vi "Test2_3b_ASIC_mezzanine_pepe.vi"(0 "Instrument VISA in":T1={"AWG VISA"="generadorpulsos", "Oscilloscope  VISA "="Oscilloscope", "Integration Board IP"="172.16.7.43", "connection ID"=refnum, "report out"=refnum, "report file path"=path "D:/CTA/Data_test/ASIC/test3a"}, 5 "quantity":i32=3, 7 "Cycles Burst":i32=10000, 9 "L1 Address":i32=17, 11 "error in":errorcluster={"status"=FALSE, "code"=0, "source"="VISA Write in Test2_3a_ASIC_fast.vi->test_sum_ASIC.vi"}, 12 "channel array":i32[](array[numeric])=[0, 1, 2, 3, 4, 5, 6]) -> (4 "Instrument VISA out":T1={"AWG VISA"="generadorpulsos", "Oscilloscope  VISA "="Oscilloscope", "Integration Board IP"="172.16.7.43", "connection ID"=refnum, "report out"=refnum, "report file path"=path "D:/CTA/Data_test/test3a"}, 15 "error out":errorcluster)   [LabVIEW 2009]
uses:
  <vilib>/Utility/NIReport.llb/NI_report.lvclass
  <vilib>/Utility/NIReport.llb/HTML/NI_HTML.lvclass
  <instrlib>/Agilent 8000 Series/Public/Configure/Configure Math (Binary Operation).vi
  <instrlib>/Agilent 81150/Agilent 81150.lvlib
  L0_Asic/L0 Asic Test Folder v9/C/Program Files/National Instruments/LabVIEW 2012/instr.lib/Agilent 8000 Series/Agilent 8000 Series.lvlib
panel:
  in  "Cycles Burst 2":i32=10000
  out "Filename Out":path
  out "appended path":path
  out "Array":i32[](array[numeric])=[2, 3, 5]
  out "points quantity":dbl=94.0
  out "appended array":dbl[](array[numeric])=[0.75, 42.0, 0.0, 63.0, 1.0, 1.069, 0.0055, 2.925838e-09, 1.2702e-11, 0.0555, 0.0035, 9.99999e+37, 9.99999e+37, 6.264189e-09, 3.2805e-11, 94.0]
  out "read buffer 3":string="V amptd(f2),1.074E+00,0,1.056E+00,1.087E+00,1.0690E+00,5.5E-03,9.4E+01,+ width(f2),2.90015E-09,0,2.90015E-09,2.95960E-09,2.925838E-09,1.2702E-11,9.4E+01,V amptd(1),5.5E-02,0,4.8E-02,6.7E-02,5.55E-02,3.5E-03,9.4E+01,+ width(f1),9.99999E+37,5,9.99999E+37,9.99999E+37,9.99999E+37,9.99999E+37,9.99999E+37,Time(f1-f2),6.26722E-09,0,6.20145E-09,6.35270E-09,6.264189E-09,3.2805E-11,9.4E+01\n"
  in  "Quantity of measurements":u32=100
  in  "Voltage":dbl[](array[numeric])=[0.05, 0.2, 0.5, 0.7, 1.0]
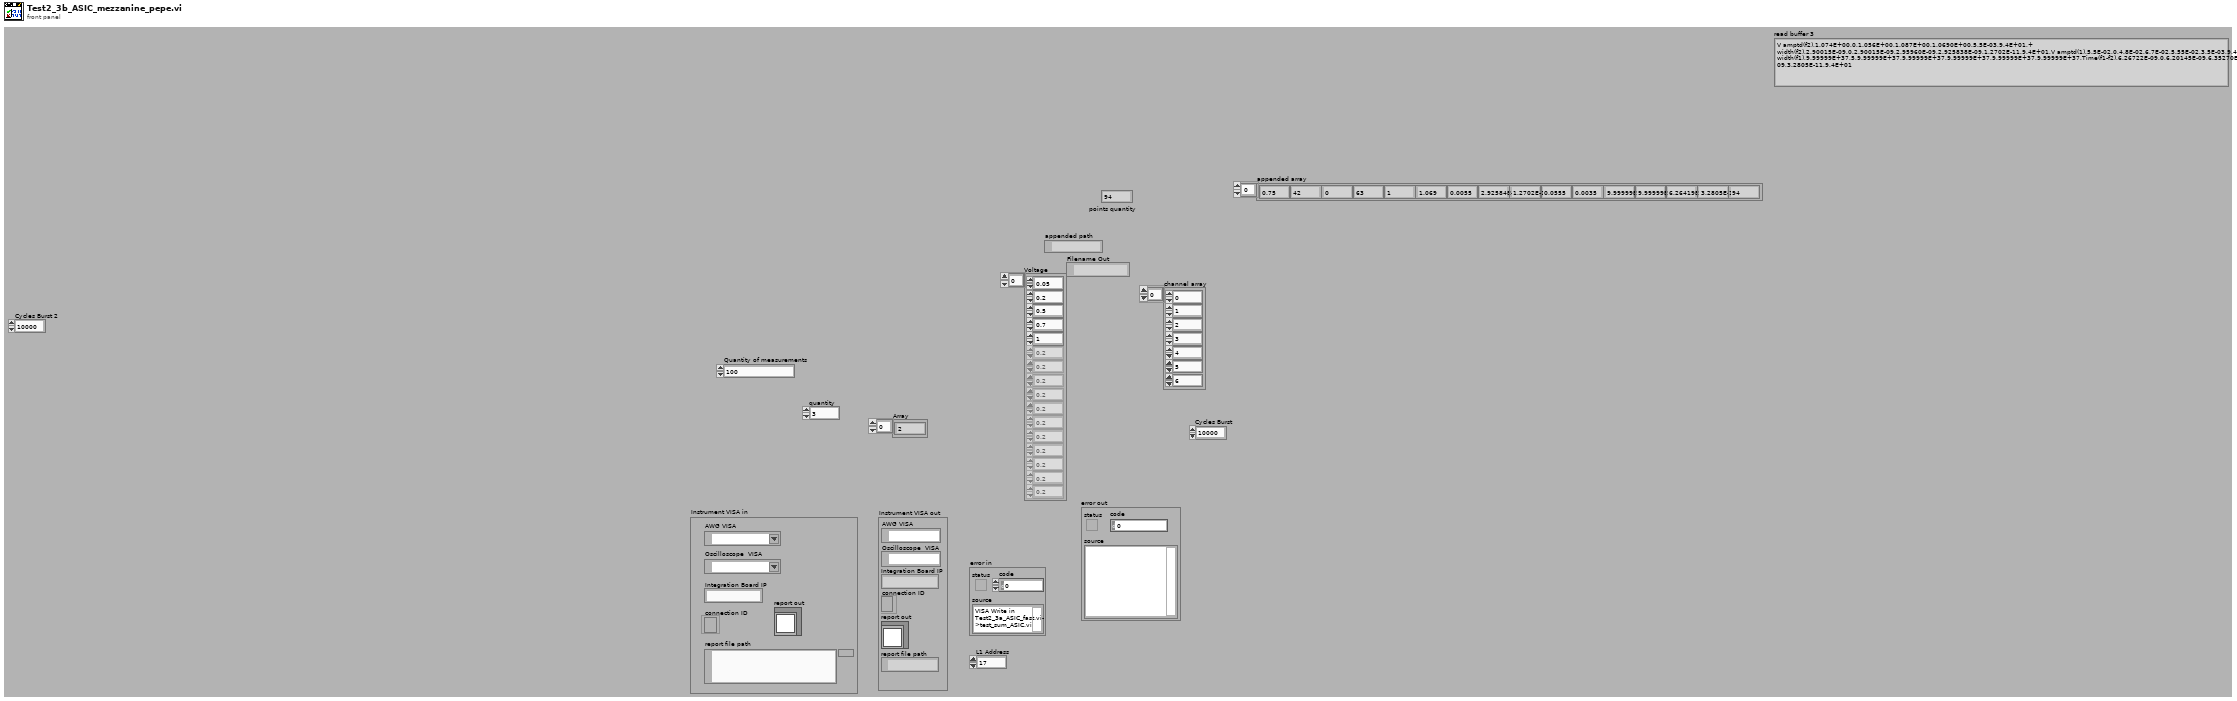
[diagram p1: front panel]
types:
  T1 = cluster{"AWG VISA":refnum<visa-resource-name>, "Oscilloscope  VISA ":refnum<visa-resource-name>, "Integration Board IP":string, "connection ID":refnum<k5>, "report out":refnum<class "NI_report.lvclass">, "report file path":path}
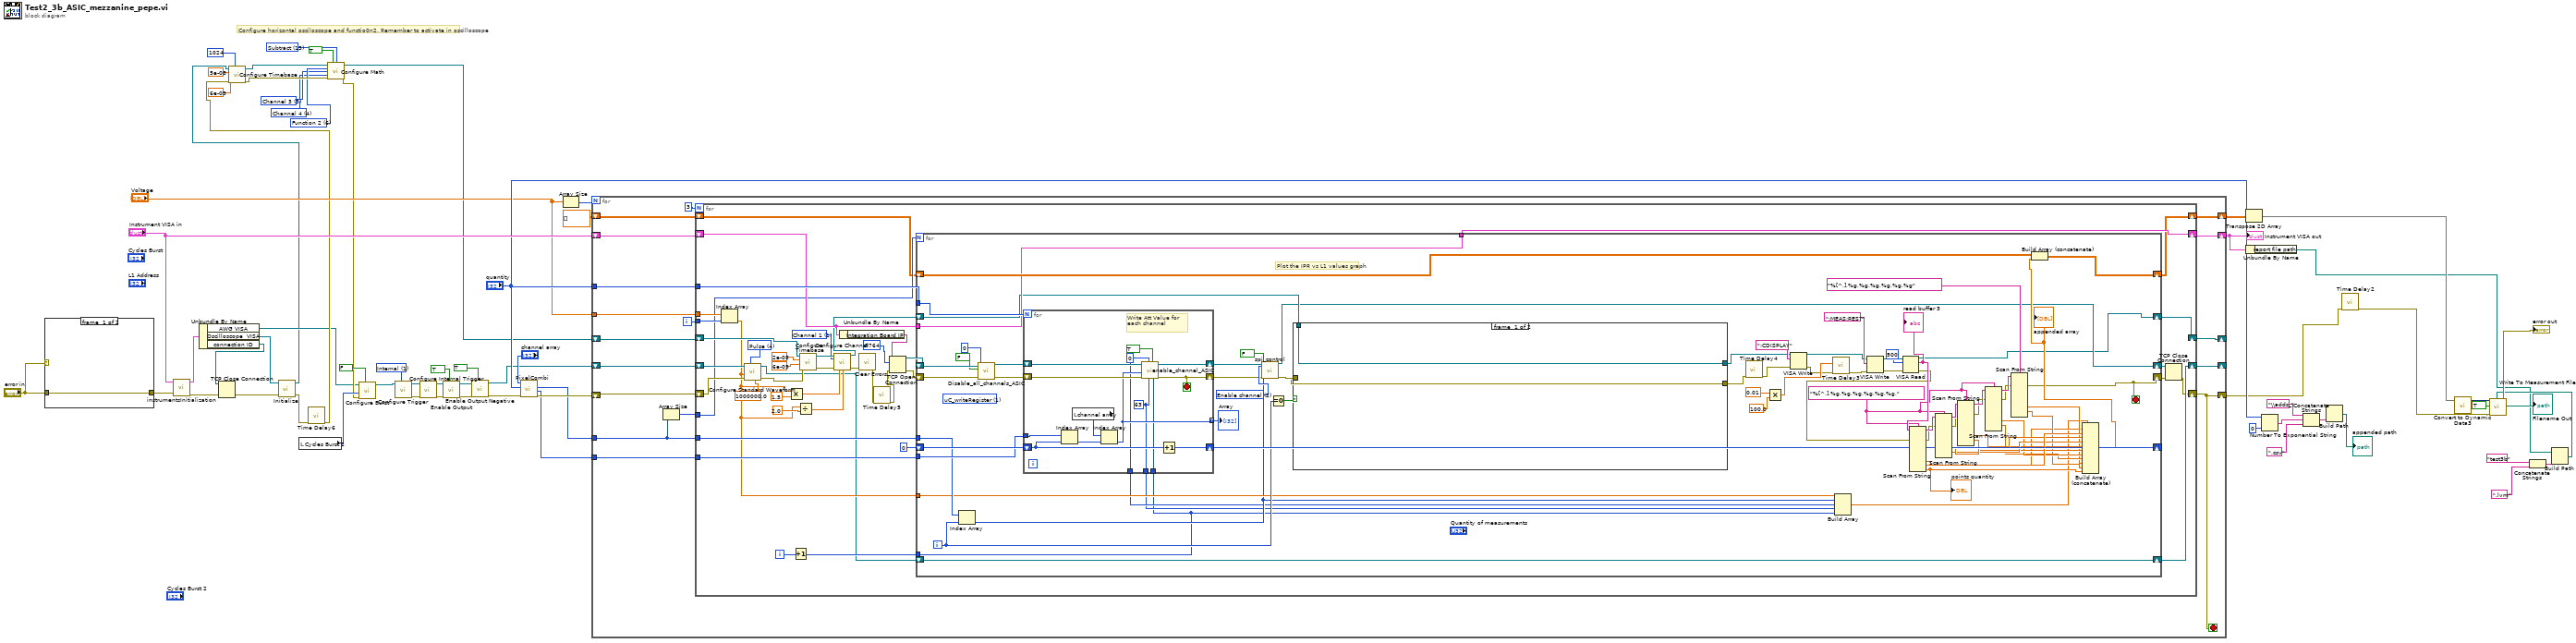
[diagram p0: block diagram]
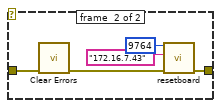
[diagram p2: hidden frame]
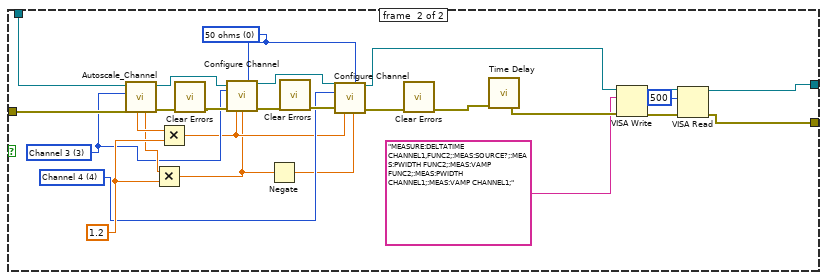
[diagram p3: hidden frame]
diagram:
  w13 = u16 6 items=["Function 1"=5, "Function 2"=6, "Function 3"=7, "Function 4"=8] ("Math Channel (5: Function 1)")
  w17 = u16 15 items=["Add"=12, "Divide"=13, "Multiply"=14, "Subtract"=15, "Common Mode"=16, "Versus"=17] ("Math Operation (12: Add)")
  w12 = 3 items=["Channel 1"=1, "Channel 2"=2, "Channel 3"=3, "Channel 4"=4] ("Channel (1: Channel 1)")
  w11 = 4 items=["Channel 1"=1, "Channel 2"=2, "Channel 3"=3, "Channel 4"=4] ("Channel (1: Channel 1)")
  w40 = u16 1 items=["Immediate", "Internal", "External", "Software Trigger Function"] ("Trigger Source (0: Immediate)")
  # "Configure horizontal osciloscope and functio0n2. Remember to activate in oscilloscope"
  n1 = case shown="No Error" "error in" {
    tunnel: "error in" -> [w66 w68]
    tunnel: [w66 w71] -> w36
    frame #0 {
    }
    frame #1 {
      n2 = call <vilib>:"Clear Errors.vi"("error in (no error)"=w68) -> ("error out"=w67:errorcluster)  [unwired: 6 in]
      n3 = call "resetboard.vi"("error in (no error)"=w67, "address"="172.16.7.43", "remote port or service name"=u16 9764) -> ("error out"=w71:errorcluster)  [unwired: 7 in, 1 out]
    }
  }
  n4 = call "instrumentsInitialization.vi"("error in"=w36, "Instrument VISA in"="Instrument VISA in") -> ("error out"=w27:errorcluster, "Instrument VISA out"=w58:T1)  [unwired: 8 in]
  n5 = Unbundle By Name(w58) -> ("AWG VISA"=w4:refnum<visa-resource-name>, "Oscilloscope  VISA"=w26:refnum<visa-resource-name>, "connection ID"=w35:refnum<k5>)
  n6 = TCP Close Connection(connection ID=w35) -> ()  [unwired: 2 in, 2 out]
  n7 = call <instrlib>:"Initialize.vi"("error in (no error)"=w27, "VISA resource name"=w26) -> ("error out"=w7:errorcluster, "VISA resource name out"=w1:refnum<visa-resource-name>)  [unwired: 8 in]
  n8 = local read "Cycles Burst 2"() -> (w8:i32)
  n9 = call "Time Delay6"("error in (no error)"=w7) -> ("error out"=w6:errorcluster)  [unwired: 10 in]
  n10 = call <instrlib>:"Configure Timebase.vi"("Record Length (1000)"=1024, "error in (no error)"=w6, "Position (0.0 s)"=6e-09, "Timebase (0.005 s)"=5e-08, "VISA resource name"=w1) -> ("error out"=w14:errorcluster, "VISA resource name out"=w15:refnum<visa-resource-name>)  [unwired: 5 in]
  n11 = call-poly <instrlib>:"Configure Math.vi"("VISA resource name"=w15, "Enable Math Channel (T:Enable)"=TRUE, "Math Operation (12: Add)"=w17, "Math Channel (5: Function 1)"=w13, "Math Operand (1: Channel 1)"=w12, "Math Operand (2: Channel 2)"=w11, "error in (no error)"=w14) -> ("VISA resource name out"=w2:refnum<visa-resource-name>, "error out"=w5:errorcluster)  [unwired: 7 in]
  n12 = call <instrlib>:"Configure Burst.vi"("Enable Burst (F: Disable)"=FALSE, "error in (no error)"=w5, "Burst Count (2)"=w8, "VISA resource name"=w4) -> ("VISA resource name out"=w3:refnum<visa-resource-name>)  [unwired: 6 in, 1 out]
  n13 = call <instrlib>:"Configure Trigger.vi"("Trigger Source (0: Immediate)"=w40, "VISA resource name"=w3) -> ("error out"=w41:errorcluster, "VISA resource name out"=w42:refnum<visa-resource-name>)  [unwired: 8 in]
  n14 = call <instrlib>:"Configure Internal Trigger.vi"("error in (no error)"=w41, "VISA resource name"=w42) -> ("error out"=w43:errorcluster, "VISA resource name out"=w44:refnum<visa-resource-name>)  [unwired: 8 in]
  n15 = call <instrlib>:"Enable Output.vi"("Enable Output (T: Enable)"=TRUE, "error in (no error)"=w43, "VISA resource name"=w44) -> ("error out"=w34:errorcluster, "VISA resource name out"=w33:refnum<visa-resource-name>)  [unwired: 7 in]
  n16 = call <instrlib>:"Enable Output Negative.vi"("Enable Output (T: Enable)"=TRUE, "error in (no error)"=w34, "VISA resource name"=w33) -> ("error out"=w32:errorcluster, "VISA resource name out"=w31:refnum<visa-resource-name>)  [unwired: 7 in]
  n17 = call "PixelCombi.vi"("error in"=w32, "quantity"="quantity", "array"="channel array") -> ("error out"=w64:errorcluster, "Channels"=w63:i32[], "Combination Array"=w62:i16[])  [unwired: 6 in]
  n18 = Array Size(array="Voltage") -> (size(s)=w59:i32)
  n19 = for {
    N: w59 -> [_]
    tunnel: w63 -> [w86]
    tunnel: w62 -> [w85]
    shift-right: [w72] -> w46
    shift-left: w64 -> [w88]
    tunnel: "Voltage" -> [w84]
    tunnel: "quantity" -> [w82]
    shift-right: [w77] -> w45
    shift-left: "Instrument VISA in" -> [w80]
    shift-right: [w76] -> w49
    shift-left: dbl[][] [] -> [w78]
    shift-right: [w73] -> _
    shift-left: w31 -> [w87]
    shift-right: [w74] -> _
    shift-left: w2 -> [w81]
    i -> [w83]
    stop <- w72 stop-if-true
    n20 = Array Size(array=w85) -> (size(s)=w79:i32)
    n21 = for {
      N: 3 -> [_]
      tunnel: w86 -> [w127]
      tunnel: w85 -> [w125]
      tunnel: w84 -> [w124]
      tunnel: w83 -> [w123]
      tunnel: w82 -> [w122]
      tunnel: w79 -> [w107]
      shift-right: [w97] -> w76
      shift-left: w78 -> [w100]
      shift-right: [w98] -> w77
      shift-left: w80 -> [w111]
      shift-right: [w92] -> w72
      shift-left: w88 -> [w129]
      shift-right: [w93] -> w73
      shift-left: w87 -> [w128]
      shift-right: [w95] -> w74
      shift-left: w81 -> [w118]
      i -> [w89]
      w114 = 1 items=["Channel 1"=1, "Channel 2"=2, "Channel 3"=3, "Channel 4"=4] ("Channel (1: Channel 1)")
      w131 = u16 4 items=["Sine", "Square", "Ramp Up", "Ramp Down", "Pulse", "Noise", "DC"] ("Waveform (0: Sine)")
      n22 = Index Array(array=w124, index=w123) -> (element=w99:dbl)
      n23 = call <instrlib>:"Configure Standard Waveform.vi"("Frequency (1000.0 Hz)"=1000000.0, "Waveform (0: Sine)"=w131, "error in (no error)"=w129, "Amplitude (1.0 Vpp)"=w99, "VISA resource name"=w128) -> ("error out"=w121:errorcluster, "VISA resource name out"=w94:refnum<visa-resource-name>)  [unwired: 5 in]
      n24 = Multiply(x=w99, y=1.5) -> (x*y=w113:dbl)
      n25 = Increment(x=w89) -> (x+1=w96:i32)
      n26 = Divide(x=w99, y=2.0) -> (x/y=w105:dbl)
      n27 = call <instrlib>:"Configure Timebase.vi"("error in (no error)"=w121, "Position (0.0 s)"=6e-09, "Timebase (0.005 s)"=2e-08, "VISA resource name"=w118) -> ("error out"=w120:errorcluster, "VISA resource name out"=w117:refnum<visa-resource-name>)  [unwired: 6 in]
      n28 = call "Configure Channel.vi"("VISA resource name"=w117, "Channel (1: Channel 1)"=w114, "error in (no error)"=w120, "Vertical Range (2.0 V)"=w113, "Vertical Offset (0.0 V)"=w105) -> ("VISA resource name out"=w104:refnum<visa-resource-name>, "error out"=w119:errorcluster)  [unwired: 9 in]
      n29 = Unbundle By Name(w111) -> ("Integration Board IP"=w109:string)
      n30 = call <vilib>:"Clear Errors.vi"("error in (no error)"=w119) -> ("error out"=w91:errorcluster)  [unwired: 6 in]
      n31 = call "Time Delay5"("error in (no error)"=w91) -> ("error out"=w90:errorcluster)  [unwired: 10 in]
      n32 = TCP Open Connection(address=w109, remote port or service name=u16 9764, error in (no error)=w90) -> (connection ID=w101:refnum<k5>, error out=w110:errorcluster)  [unwired: 2 in]
      n33 = for {
        N: w107 -> [_]
        tunnel: w125 -> [w199]
        tunnel: w127 -> [w200]
        shift-right: [w201] -> _
        shift-left: i16 0 ("element") -> [w202]
        shift-right: [w146] -> w103
        shift-left: w110 -> [w192]
        tunnel: w111 -> [w187]
        tunnel: w122 -> [w198]
        tunnel: [w187] -> w98
        shift-right: [w193] -> w97
        shift-left: w100 -> [w194]
        shift-right: [w147] -> w102
        shift-left: w101 -> [w145]
        tunnel: w99 -> [w142]
        tunnel: w96 -> [w137]
        shift-right: [w136] -> w95
        shift-left: w104 -> [w185]
        shift-right: [w135] -> w93
        shift-left: w94 -> [w135]
        i -> [w183]
        stop <- w146 stop-if-true
        w168 = "%[^,],%g,%g,%g,%g,%g,%g," ("format string")
        w191 = u16 2 items=["Attenuation", "Clipping", "Enable channel", "Delay line", "ASIC"] ("Device")
        (unwired) u16 1 items=["sendCommand"=9, "FPGA_writeRegister"=3, "FPGA_readRegister"=2, "uC_writeRegister"=1, "uC_readRegister"=0] ("Action")
        # "Plot the IPR vs L1 values graph"
        n34 = Index Array(array=w199, index=w183) -> (element=w141:i16)
        n35 = call "Disable_all_channels_ASIC.vi"("error in"=w192, "id_in"=0 ("Data"), "Clip_en_b"=FALSE, "connection ID"=w145) -> ("error out"=w196:errorcluster, "connection ID out"=w195:refnum<k5>)  [unwired: 5 in, 1 out]
        n36 = for {
          N: w198 -> [_]
          shift-right: [w244] -> w201
          shift-left: w202 -> [w245]
          tunnel: w200 -> [w243]
          shift-right: [w240] -> w189
          shift-left: w196 -> [w239]
          shift-right: [w237] -> w188
          shift-left: w195 -> [w238]
          tunnel: [w236] -> w144 mode=indexing
          tunnel: [w235] -> w140
          tunnel: [w234] -> w139
          tunnel: w137 -> [w233]
          stop <- w240 stop-if-true
          w235 = u32 0 ("Att gain")
          w234 = u32 63 ("Ib_clipVb")
          # "Write Att Value for each channel"
          n37 = Index Array(array=w243, index=w245) -> (element=w241:i32)
          n38 = local read "channel array"() -> (w242:i32[])
          n39 = Index Array(array=w242, index=w241) -> (element=w236:i32)
          n40 = call "enable_channel_ASIC.vi"("Clip_sel_b"=w233, "maj/sum"=TRUE, "Ib_clipVb"=w234, "Att gain"=w235, "error in"=w239, "Channel"=w236, "connection ID"=w238) -> ("error out"=w240:errorcluster, "connection ID out"=w237:refnum<k5>)  [unwired: 2 in, 1 out]
          n41 = Increment(x=w245) -> (x+1=w244:i16)
        }
        "Array" <- w144
        n42 = call "spi_control.vi"("connection ID"=w188, "Device"=w191, "Read/#write"=FALSE, "Data"=w141, "error out 3"=w189) -> ("connection ID out"=w147:refnum<k5>, "error out 2"=w186:errorcluster)  [unwired: 7 in, 6 out]
        n43 = Equal To 0?(x=w183) -> (x = 0?=w184:bool)
        n44 = case shown="True" w184 {
          tunnel: [w204 w211] -> w132
          tunnel: w186 -> [w204 w217]
          tunnel: w185 -> [w203 w218]
          tunnel: [w203 w220] -> w150
          frame #0 {
          }
          frame #1 {
            w221 = u32 0 items=["50 ohms", "1 Mohms"] ("Input Impedance (1: 1 Mohms)")
            w209 = 3 items=["Channel 1"=1, "Channel 2"=2, "Channel 3"=3, "Channel 4"=4] ("Channel (1: Channel 1)")
            w208 = 4 items=["Channel 1"=1, "Channel 2"=2, "Channel 3"=3, "Channel 4"=4] ("Channel (1: Channel 1)")
            w214 = 1.2 ("y")
            n45 = call "Autoscale_Channel.vi"("error in"=w217, "Channel"=w209, "VISA resource name"=w218) -> ("error out"=w228:errorcluster, "VISA resource name out"=w231:refnum<visa-resource-name>, "Offset"=w210:dbl, "VerticalRange"=w225:dbl)  [unwired: 5 in]
            n46 = Multiply(x=w210, y=w214) -> (x*y=w206:dbl)
            n47 = Multiply(x=w225, y=w214) -> (x*y=w207:dbl)
            n48 = call <vilib>:"Clear Errors.vi"("error in (no error)"=w228) -> ("error out"=w229:errorcluster)  [unwired: 6 in]
            n49 = call "Configure Channel.vi"("VISA resource name"=w231, "Input Impedance (1: 1 Mohms)"=w221, "Channel (1: Channel 1)"=w209, "error in (no error)"=w229, "Vertical Range (2.0 V)"=w207, "Vertical Offset (0.0 V)"=w206) -> ("VISA resource name out"=w226:refnum<visa-resource-name>, "error out"=w230:errorcluster)  [unwired: 8 in]
            n50 = Negate(x=w206) -> (-x=w205:dbl)
            n51 = call <vilib>:"Clear Errors.vi"("error in (no error)"=w230) -> ("error out"=w219:errorcluster)  [unwired: 6 in]
            n52 = call "Configure Channel.vi"("VISA resource name"=w226, "Input Impedance (1: 1 Mohms)"=w221, "Channel (1: Channel 1)"=w208, "error in (no error)"=w219, "Vertical Range (2.0 V)"=w207, "Vertical Offset (0.0 V)"=w205) -> ("VISA resource name out"=w215:refnum<visa-resource-name>, "error out"=w227:errorcluster)  [unwired: 8 in]
            n53 = call <vilib>:"Clear Errors.vi"("error in (no error)"=w227) -> ("error out"=w216:errorcluster)  [unwired: 6 in]
            n54 = call "Time Delay"("error in (no error)"=w216) -> ("error out"=w213:errorcluster)  [unwired: 10 in]
            n55 = VISA Write(VISA resource name=w215, write buffer="MEASURE:DELTATIME CHANNEL1,FUNC2;:MEAS:SOURCE?;:MEAS:PWIDTH FUNC2;:MEAS:VAMP FUNC2;:MEAS:PWIDTH CHANNEL1;:MEAS:VAMP CHANNEL1;", error in (no error)=w213) -> (VISA resource name out=w224:refnum<visa-resource-name>, error out=w223:errorcluster)  [unwired: 1 out]
            n56 = VISA Read(VISA resource name=w224, byte count=u32 500, error in (no error)=w223) -> (VISA resource name out=w220:refnum<visa-resource-name>, error out=w211:errorcluster)  [unwired: 2 out]
          }
        }
        n57 = call "Time Delay4"("error in (no error)"=w132) -> ("error out"=w133:errorcluster)  [unwired: 10 in]
        n58 = Multiply(x=0.01, y=100.0) -> (x*y=w175:dbl)
        n59 = VISA Write(VISA resource name=w150, write buffer=":CDISPLAY", error in (no error)=w133) -> (VISA resource name out=w153:refnum<visa-resource-name>, error out=w151:errorcluster)  [unwired: 1 out]
        n60 = call "Time Delay3"("error in (no error)"=w151, "Delay Time (s)"=w175) -> ("error out"=w174:errorcluster)  [unwired: 9 in]
        n61 = Build Array(w142, w141, w140, w139, w137) -> (w138:dbl[])
        n62 = VISA Write(VISA resource name=w153, write buffer=":MEAS:RES?", error in (no error)=w174) -> (VISA resource name out=w182:refnum<visa-resource-name>, error out=w181:errorcluster)  [unwired: 1 out]
        n63 = VISA Read(VISA resource name=w182, byte count=u32 500, error in (no error)=w181) -> (VISA resource name out=w136:refnum<visa-resource-name>, read buffer=w178:string, error out=w158:errorcluster)  [unwired: 1 out]
        "read buffer 3" <- w178
        n64 = Scan From String(format string=w168, input string=w178, error in=w158) -> (remaining string=w172:string, error out=w154:errorcluster, output 5=w143:dbl, output 6=w173:dbl, output 7=w159:dbl)  [unwired: 12 in, 1 out]
        "points quantity" <- w159
        n65 = Scan From String(format string=w168, input string=w172, error in=w154) -> (remaining string=w169:string, error out=w155:errorcluster, output 5=w166:dbl, output 6=w165:dbl)  [unwired: 13 in, 1 out]
        n66 = Scan From String(format string=w168, input string=w169, error in=w155) -> (remaining string=w170:string, error out=w156:errorcluster, output 5=w164:dbl, output 6=w163:dbl)  [unwired: 13 in, 1 out]
        n67 = Scan From String(format string=w168, input string=w170, error in=w156) -> (remaining string=w171:string, error out=w157:errorcluster, output 5=w162:dbl, output 6=w161:dbl)  [unwired: 13 in, 1 out]
        n68 = Scan From String(format string="%[^,],%g,%g,%g,%g,%g,%g", input string=w171, error in=w157) -> (error out=w146:errorcluster, output 5=w149:dbl, output 6=w160:dbl)  [unwired: 13 in, 2 out]
        n69 = Build Array (concatenate)(w138, w143, w173, w166, w165, w164, w163, w162, w161, w149, w160, w159) -> (w148:dbl[])
        "appended array" <- w148
        n70 = Build Array (concatenate)(w194, w148) -> (w193:dbl[][])
      }
      n71 = TCP Close Connection(connection ID=w102, error in (no error)=w103) -> (error out=w92:errorcluster)  [unwired: 1 in, 1 out]
    }
  }
  "Instrument VISA out" <- w45
  n72 = Transpose 2D Array(2D array=w49) -> (transposed array=w38:dbl[][])
  n73 = Unbundle By Name(w45) -> ("report file path"=w20:path)
  n74 = Number To Exponential String(number="quantity", precision (6)=i16 0) -> (E-format string=w53:string)  [unwired: 2 in]
  n75 = Concatenate Strings("\\adds_" ("string"), w53, ".csv" ("name or relative path")) -> (w56:string)
  n76 = Build Path(name or relative path=w56) -> (appended path=→"appended path":path)  [unwired: 1 in]
  n77 = call "Time Delay2"("error in (no error)"=w46) -> ("error out"=w60:errorcluster)  [unwired: 10 in]
  n78 = call "Convert to Dynamic Data3"("2D Array"=w38) -> ("Dynamic Data Type"=w39:dynamicdata)  [unwired: 3 in]
  n79 = Concatenate Strings("test3b" ("string"), ".lvm" ("name or relative path")) -> (w24:string)
  n80 = Build Path(base path=w20, name or relative path=w24) -> (appended path=w21:path)
  n81 = call "Write To Measurement File"("Signals"=w39, "Enable"=TRUE, "error in (no error)"=w60, "Filename"=w21) -> ("Filename Out"=→"Filename Out":path, "error out"=→"error out":errorcluster)  [unwired: 13 in, 1 out]
